vi "Exemple_Extraction_TfidfTransformer.vi"() -> ()   [LabVIEW 2020]
uses:
  Objet/6 - Datasets Transformation/6.2 - Feature extraction/TfidfTransformer/TfidfTransformer.lvclass
panel:
  in  "Type X":enum16{"Array", "Sparse"}(ring)=enum."Sparse"
  in  "y":string[][](array[string])
  in  "X":string[][](array[string])=[["0", "1", "0.5773502691896258"], ["0", "0", "0.5773502691896258"], ["0", "2", "0.5773502691896258"], ["1", "1", "0.5773502691896258"], ["1", "0", "0.5773502691896258"], ["1", "2", "0.5773502691896258"], ["2", "1", "0.5773502691896258"], ["2", "0", "0.5773502691896258"], ["2", "2", "0.5773502691896258"], ["3", "1", "0.5773502691896258"], ["3", "0", "0.5773502691896258"], ["3", "2", "0.5773502691896258"]]
  in  "TfidfTransformer":T1={"norm"="l2", "use_idf"=TRUE, "smooth_idf"=TRUE, "sublinear_tf"=FALSE}
  out "Data":T2
  out "error out":errorcluster caption="sortie d'erreur"
  in  "error in":errorcluster caption="entrée d'erreur"
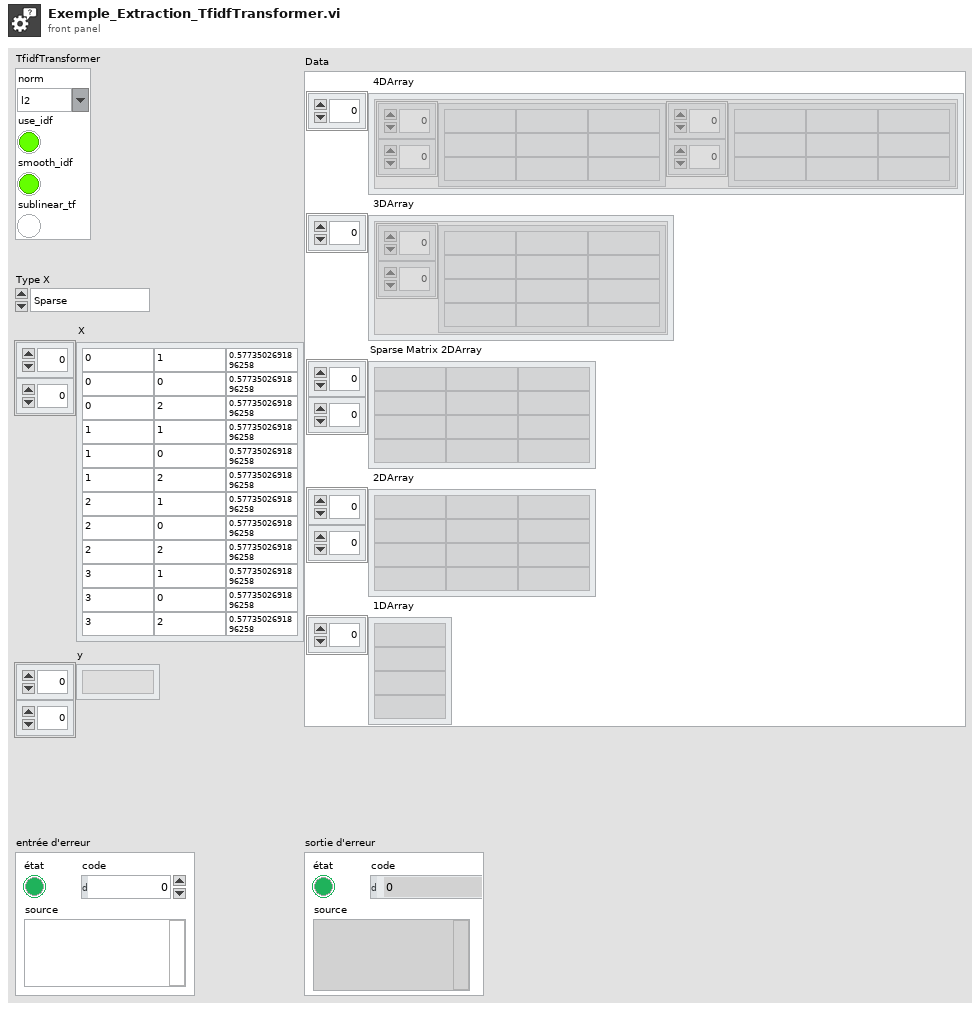
[diagram p1: front panel]
types:
  T1 = cluster{"norm":string, "use_idf":bool, "smooth_idf":bool, "sublinear_tf":bool}
  T2 = cluster{" 4DArray":cluster{"1":string[][], "2":string[][]}[], " 3DArray":cluster{"Tableau":string[][]}[], "Sparse Matrix 2DArray":string[][], " 2DArray":string[][], " 1DArray":string[]}
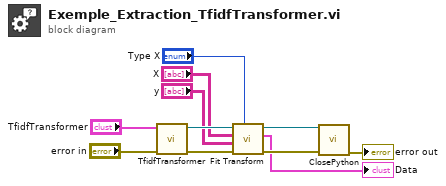
[diagram p0: block diagram]
diagram:
  n1 = call "TfidfTransformer.vi"("error in"="error in", "TfidfTransformer"="TfidfTransformer") -> ("error out"=w8:errorcluster, "TfidfTransformer.lvclass"=w9:refnum<class "TfidfTransformer.lvclass">)  [unwired: 8 in]
  n2 = call-dynamic "Fit Transform.vi"("Type X"="Type X", "error in (no error)"=w8, "y"="y", "X"="X", "TfidfTransformer.lvclass"=w9) -> ("error out"=w4:errorcluster, "Data"=→"Data":T2, "TfidfTransformer.lvclass"=w5:refnum<class "TfidfTransformer.lvclass">)  [unwired: 4 in]
  n3 = call-dynamic "ClosePython.vi"("error in (no error)"=w4, "Scikit-learn en entrée"=w5) -> ("error out"=→"error out":errorcluster)  [unwired: 8 in, 1 out]
